vi "CC Quad Image Viewer.vi"(11 "Files":path[](array[path])) -> ()   [LabVIEW 2024]
uses:
  <vilib>/Utility/miscctls.llb/LVCursorListTypeDef.ctl
panel:
  in  "Transpose 1":bool
  out "Detector 1":sgl[][](graph)
  in  "Transpose 2":bool
  out "Detector 2":sgl[][](graph)
  in  "Transpose 3":bool
  out "Detector 3":sgl[][](graph)
  in  "Transpose 4":bool
  out "Detector 4":sgl[][](graph)
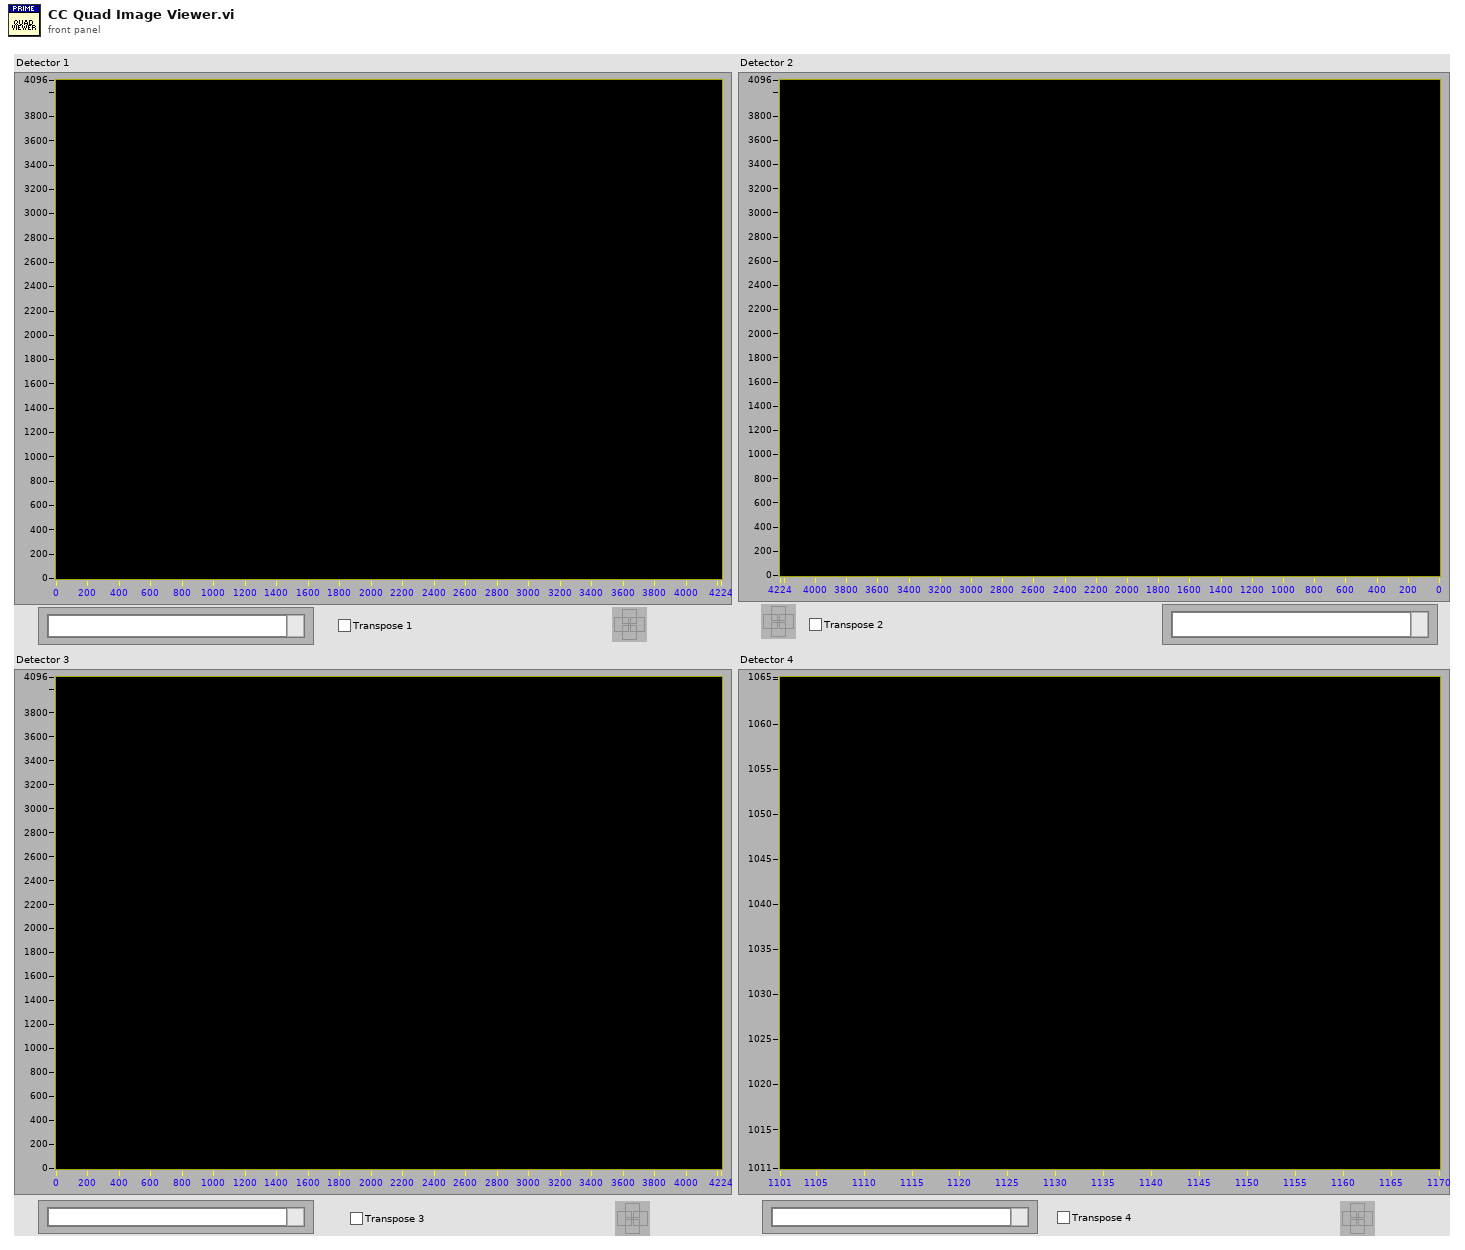
[diagram p1: front panel]
types:
  T1 = cluster{"state":refnum<user-event>, "plots":refnum<vi>[]}
  T2 = typedef "LVCursorListTypeDef.ctl" = cluster{"Name":string, "Color":u32, "Style":u8, "Point Style":u8, "Name Visible":bool, "Allow Drag":bool, "Cursor Mode":u32, "Plot":i32, "Index":i32, "Position":cluster{"X":dbl, "Y":dbl}, "X Scale":u32, "Y Scale":u32, "Watch Plots":i32[], "Watch All Plots":bool, "Plot Area":i32, "Label Offset":cluster{"X":dbl, "Y":dbl}}[]
  T3 = typedef "LVRectTypeDef.ctl" = cluster{"Left":i16, "Top":i16, "Right":i16, "Bottom":i16}
  T4 = typedef "CC cluster  Viewer Image Order.ctl" = cluster{"Top Left":i32, "Top Right":i32, "Bottom Left":i32, "Bottom Right":i32}
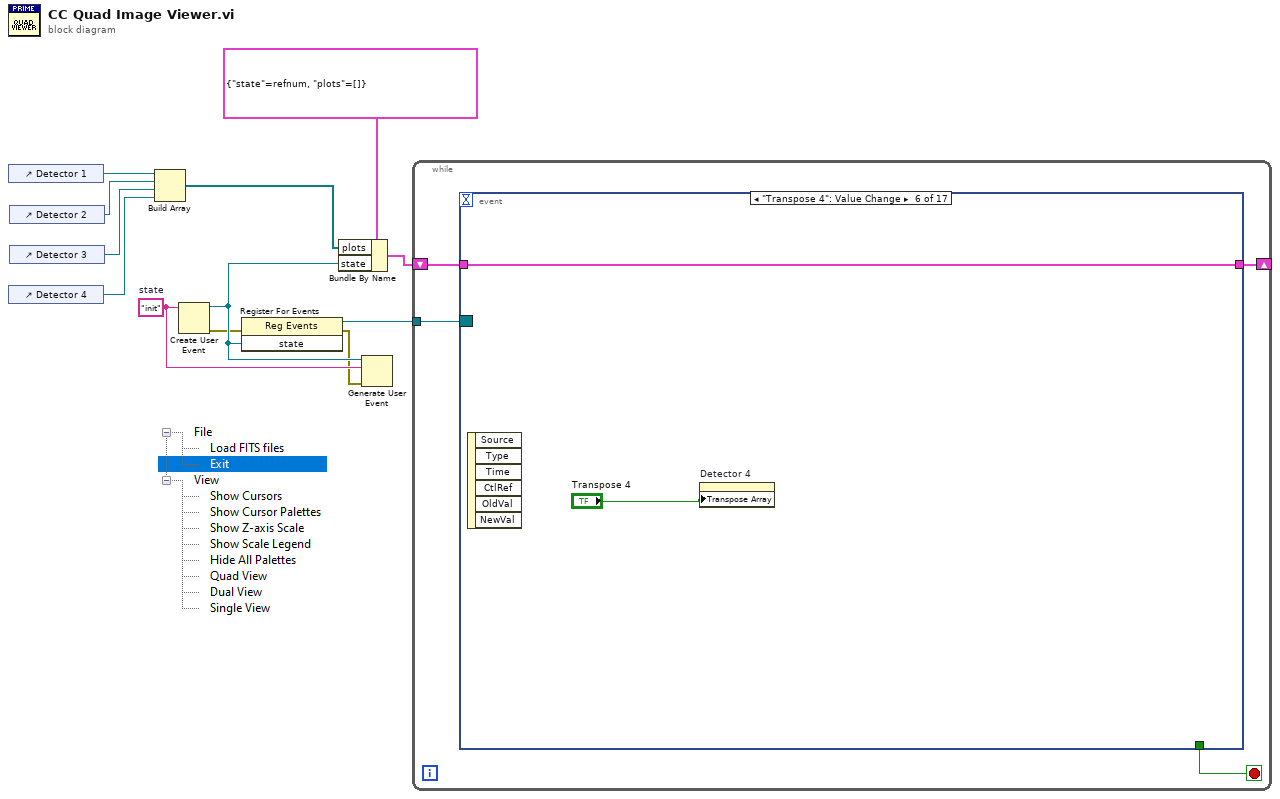
[diagram p0: block diagram]
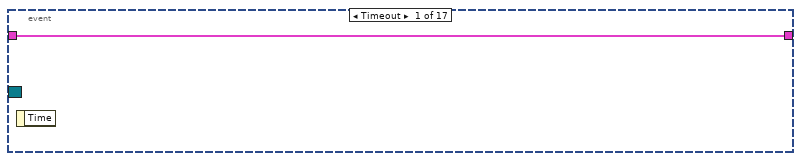
[diagram p2: hidden frame]
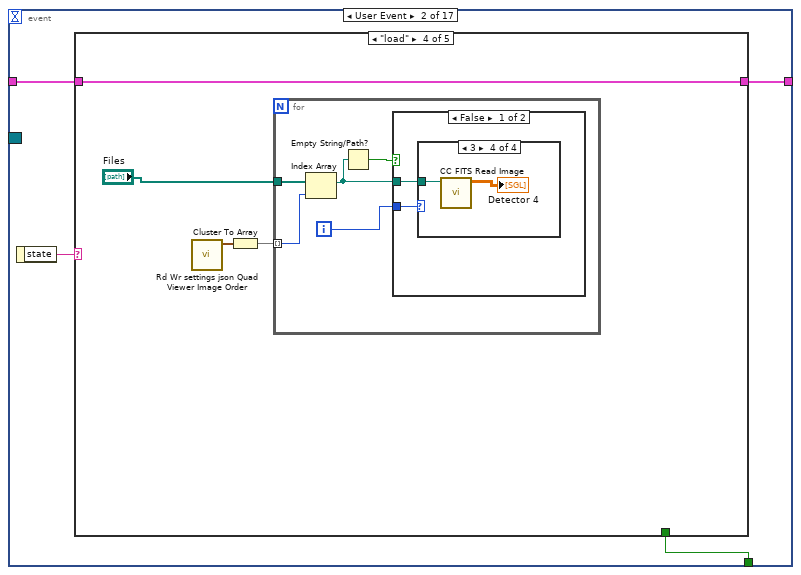
[diagram p3: hidden frame]
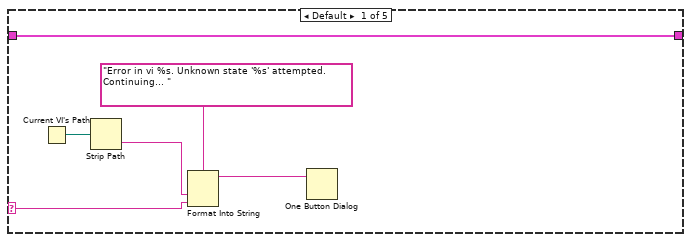
[diagram p4: hidden frame]
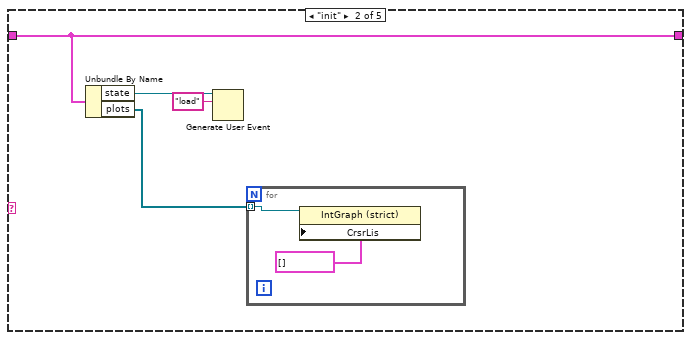
[diagram p5: hidden frame]
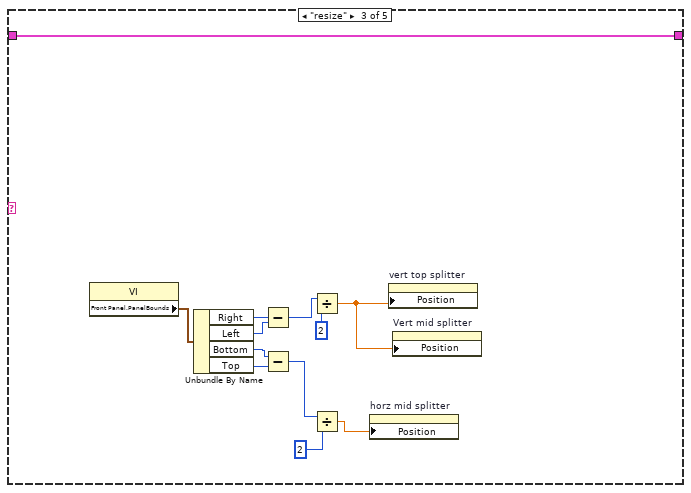
[diagram p6: hidden frame]
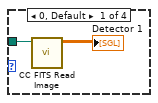
[diagram p7: hidden frame]
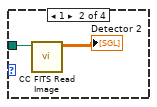
[diagram p8: hidden frame]
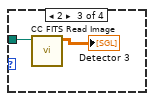
[diagram p9: hidden frame]
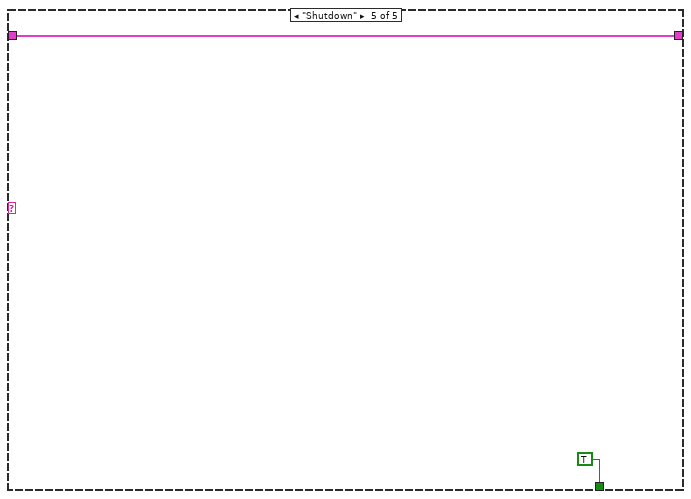
[diagram p11: hidden frame]
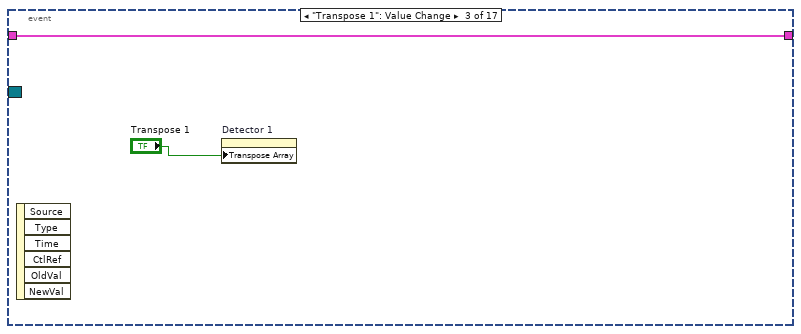
[diagram p12: hidden frame]
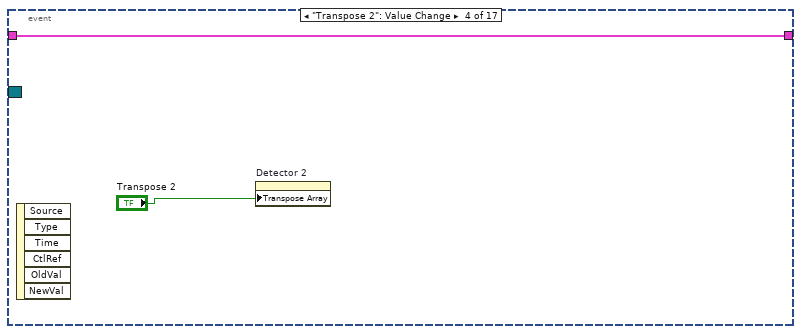
[diagram p13: hidden frame]
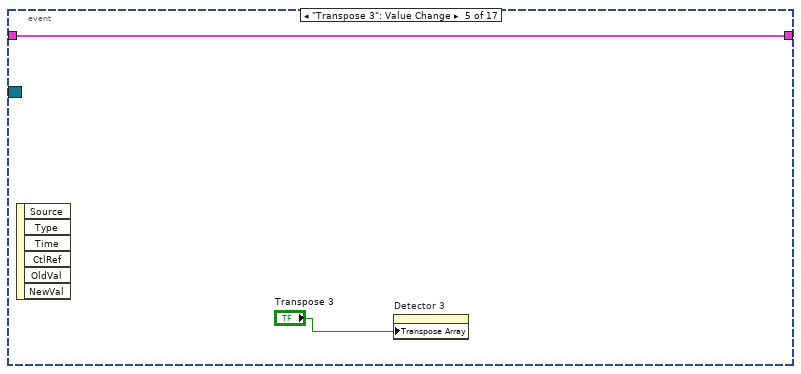
[diagram p14: hidden frame]
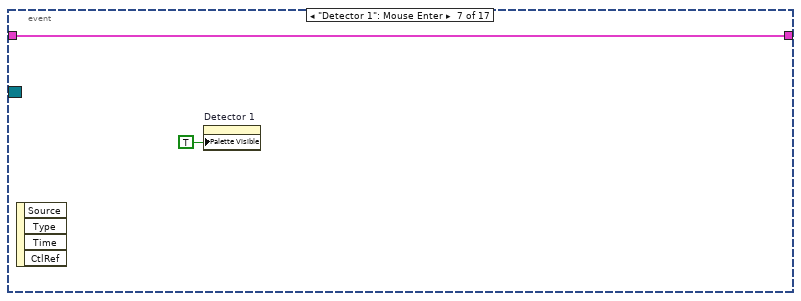
[diagram p15: hidden frame]
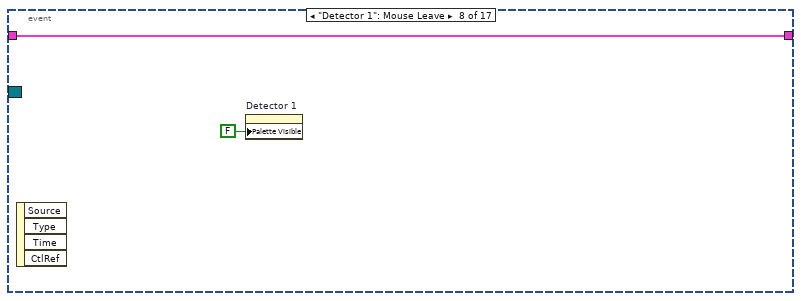
[diagram p16: hidden frame]
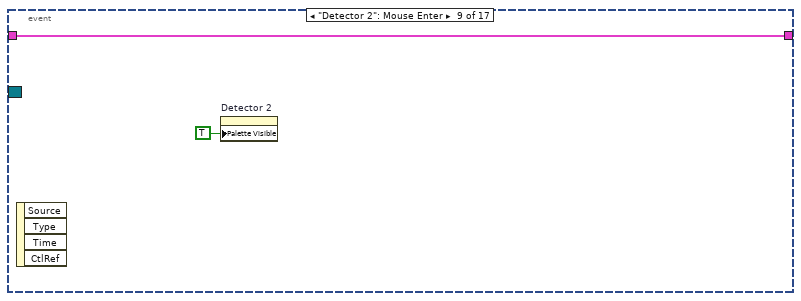
[diagram p17: hidden frame]
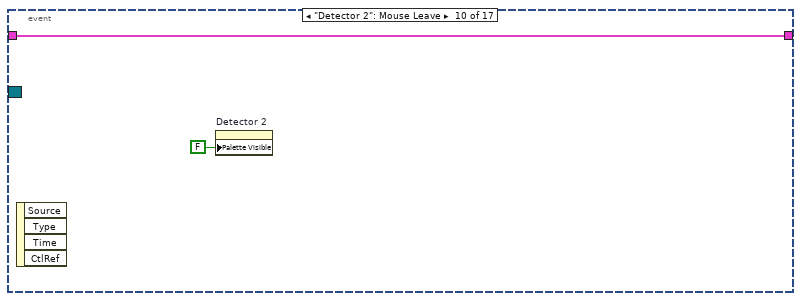
[diagram p18: hidden frame]
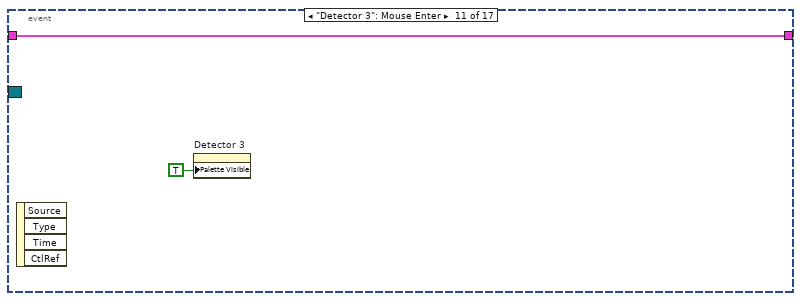
[diagram p19: hidden frame]
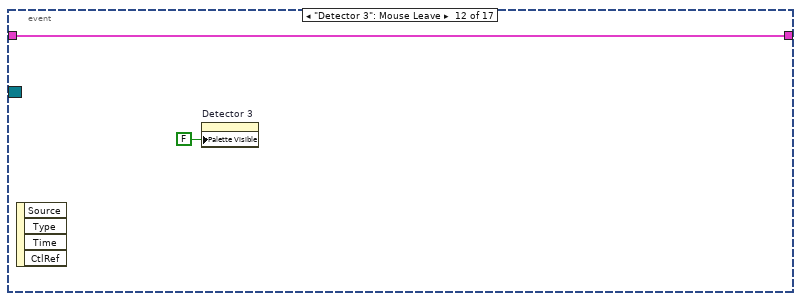
[diagram p20: hidden frame]
diagram:
  w8 = "init"  # state
  n1 = control-ref of="Detector 1"() -> (w5:refnum<vi>)
  n2 = control-ref of="Detector 4"() -> (w2:refnum<vi>)
  n3 = control-ref of="Detector 2"() -> (w4:refnum<vi>)
  n4 = control-ref of="Detector 3"() -> (w3:refnum<vi>)
  n5 = Build Array(w5, w4, w3, w2) -> (w1:refnum<vi>[])
  n6 = Create User Event(user event datatype=w8) -> (user event=w10:refnum<user-event>, error out=w6:errorcluster)  [unwired: 1 in]
  n7 = register-events(error in=w6, w10) -> (reference out=w9:refnum<event-registration>, error out=w7:errorcluster)  [unwired: 1 in]
  n8 = Bundle By Name(cluster=T1 {"state"=refnum, "plots"=[]}, "plots"=w1, "state"=w10) -> (w11:T1)
  n9 = Generate User Event(user event=w10, event data cluster=w8, error in=w7) -> ()  [unwired: 1 in, 2 out]
  n10 = while {
    tunnel: w9 -> [w16]
    shift-right: [w14] -> _
    shift-left: w11 -> [w15]
    stop <- w13 stop-if-true
    n11 = event shown="[5] \"Transpose 4\": Value Change" {
      selector: w16 -> [_ _ _ _ _ _ _ _ _ _ _ _ _ _ _ _ _]
      dyn-events: _ -> [_ _ _ _ _ _ _ _ _ _ _ _ _ _ _ _ _]
      timeout: _ -> [_ _ _ _ _ _ _ _ _ _ _ _ _ _ _ _ _]
      tunnel: w15 -> [w17 w20 w68 w70 w72 w74 w76 w78 w80 w82 w84 w86 w88 w90 w94 w151 w155]
      tunnel: [w17 w19 w68 w70 w72 w74 w76 w78 w80 w82 w84 w86 w88 w90 w94 w151 w155] -> w14
      tunnel: [_ w18 _ _ _ _ _ _ _ _ _ _ _ _ _ _ _] -> w13
      event Timeout {
        n12 = event-data() -> ()  [unwired: 1 in, 1 out]
      }
      event User Event {
        n13 = event-data() -> ("state"=w21:string)  [unwired: 1 in]
        n14 = case shown="\"load\"" w21 {
          selector: w21 -> [w26 _ _ _ _]
          tunnel: w20 -> [w22 w31 w45 w49 w66]
          tunnel: [w22 w31 w45 w49 w66] -> w19
          tunnel: [_ _ _ _ TRUE] -> w18
          frame Default {
            n15 = Current VI's Path() -> (path=w25:path)
            n16 = Strip Path(path=w25) -> (name=w24:string)  [unwired: 1 out]
            n17 = Format Into String(format string="Error in vi %s. Unknown state '%s' attempted. Continuing... ", w24, w26) -> (resulting string=w23:string)  [unwired: 2 in, 1 out]
            n18 = One Button Dialog(message=w23) -> ()  [unwired: 1 in, 1 out]
          }
          frame "init" {
            n19 = Unbundle By Name(w31) -> ("state"=w30:refnum<user-event>, "plots"=w28:refnum<vi>[])
            n20 = Generate User Event(user event=w30, event data cluster="load" ("event data")) -> ()  [unwired: 2 in, 2 out]
            n21 = for {
              tunnel: w28 -> [w33] mode=indexing
              n22 = property class="IntGraph (strict)"(reference=w33, "CrsrLis"=T2 [] ("Cursor List")) -> ()  [unwired: 1 in, 2 out]
            }
          }
          frame "resize" {
            n23 = property class="VI"() -> ("Front Panel.PanelBounds"=w42:T3)  [unwired: 2 in, 2 out]
            n24 = Unbundle By Name(w42) -> ("Right"=w39:i16, "Left"=w38:i16, "Bottom"=w35:i16, "Top"=w36:i16)
            n25 = Subtract(x=w39, y=w38) -> (x-y=w37:i16)
            n26 = Subtract(x=w35, y=w36) -> (x-y=w34:i16)
            n27 = Divide(x=w37, y=2) -> (x/y=w41:dbl)
            n28 = Divide(x=w34, y=2) -> (x/y=w40:dbl)
            n29 = property on="horz mid splitter" class="Splitter"("Position"=w40) -> ()  [unwired: 2 in, 2 out]
            n30 = property on="vert top splitter" class="Splitter"("Position"=w41) -> ()  [unwired: 2 in, 2 out]
            n31 = property on="Vert mid splitter" class="Splitter"("Position"=w41) -> ()  [unwired: 2 in, 2 out]
          }
          frame "load" {
            n32 = call "Rd Wr settings json Quad Viewer Image Order.vi"() -> ("Image Order"=w47:T4)  [unwired: 10 in, 1 out]
            n33 = Cluster To Array(cluster=w47) -> (array=w46:i32[])
            n34 = for {
              tunnel: "Files" -> [w53]
              tunnel: w46 -> [w52] mode=indexing
              i -> [w54]
              n35 = Index Array(array=w53, index=w52) -> (element=w51:path)
              n36 = Empty String/Path?(string/path=w51) -> (empty?=w50:bool)
              n37 = case shown="False" w50 {
                tunnel: w54 -> [w56 _]
                tunnel: w51 -> [w55 _]
                frame False {
                  n38 = case shown="3" w56 {
                    tunnel: w55 -> [w58 w60 w62 w64]
                    frame 0, Default {
                      n39 = call "CC FITS Read Image.vi"("FITS File Path"=w58) -> ("Image"=→"Detector 1":sgl[][])  [unwired: 9 in, 1 out]
                    }
                    frame 1 {
                      n40 = call "CC FITS Read Image.vi"("FITS File Path"=w60) -> ("Image"=→"Detector 2":sgl[][])  [unwired: 9 in, 1 out]
                    }
                    frame 2 {
                      n41 = call "CC FITS Read Image.vi"("FITS File Path"=w62) -> ("Image"=→"Detector 3":sgl[][])  [unwired: 9 in, 1 out]
                    }
                    frame 3 {
                      n42 = call "CC FITS Read Image.vi"("FITS File Path"=w64) -> ("Image"=→"Detector 4":sgl[][])  [unwired: 9 in, 1 out]
                    }
                  }
                }
                frame True {
                }
              }
            }
          }
          frame "Shutdown" {
          }
        }
      }
      event "Transpose 1": Value Change {
        n43 = event-data() -> ()  [unwired: 1 in, 6 out]
        n44 = property on="Detector 1" class="IntGraph (strict)"("Transpose Array"="Transpose 1") -> ()  [unwired: 2 in, 2 out]
      }
      event "Transpose 2": Value Change {
        n45 = event-data() -> ()  [unwired: 1 in, 6 out]
        n46 = property on="Detector 2" class="IntGraph (strict)"("Transpose Array"="Transpose 2") -> ()  [unwired: 2 in, 2 out]
      }
      event "Transpose 3": Value Change {
        n47 = event-data() -> ()  [unwired: 1 in, 6 out]
        n48 = property on="Detector 3" class="IntGraph (strict)"("Transpose Array"="Transpose 3") -> ()  [unwired: 2 in, 2 out]
      }
      event "Transpose 4": Value Change {
        n49 = event-data() -> ()  [unwired: 1 in, 6 out]
        n50 = property on="Detector 4" class="IntGraph (strict)"("Transpose Array"="Transpose 4") -> ()  [unwired: 2 in, 2 out]
      }
      event "Detector 1": Mouse Enter {
        n51 = event-data() -> ()  [unwired: 1 in, 4 out]
        n52 = property on="Detector 1" class="IntGraph (strict)"("Palette Visible"=TRUE ("Palette:Visible")) -> ()  [unwired: 2 in, 2 out]
      }
      event "Detector 1": Mouse Leave {
        n53 = event-data() -> ()  [unwired: 1 in, 4 out]
        n54 = property on="Detector 1" class="IntGraph (strict)"("Palette Visible"=FALSE ("Palette:Visible")) -> ()  [unwired: 2 in, 2 out]
      }
      event "Detector 2": Mouse Enter {
        n55 = event-data() -> ()  [unwired: 1 in, 4 out]
        n56 = property on="Detector 2" class="IntGraph (strict)"("Palette Visible"=TRUE ("Palette:Visible")) -> ()  [unwired: 2 in, 2 out]
      }
      event "Detector 2": Mouse Leave {
        n57 = event-data() -> ()  [unwired: 1 in, 4 out]
        n58 = property on="Detector 2" class="IntGraph (strict)"("Palette Visible"=FALSE ("Palette:Visible")) -> ()  [unwired: 2 in, 2 out]
      }
      event "Detector 3": Mouse Enter {
        n59 = event-data() -> ()  [unwired: 1 in, 4 out]
        n60 = property on="Detector 3" class="IntGraph (strict)"("Palette Visible"=TRUE ("Palette:Visible")) -> ()  [unwired: 2 in, 2 out]
      }
      event "Detector 3": Mouse Leave {
        n61 = event-data() -> ()  [unwired: 1 in, 4 out]
        n62 = property on="Detector 3" class="IntGraph (strict)"("Palette Visible"=FALSE ("Palette:Visible")) -> ()  [unwired: 2 in, 2 out]
      }
      event "Detector 4": Mouse Enter {
        n63 = event-data() -> ()  [unwired: 1 in, 4 out]
        n64 = property on="Detector 4" class="IntGraph (strict)"("Palette Visible"=TRUE ("Palette:Visible")) -> ()  [unwired: 2 in, 2 out]
      }
      event "Detector 4": Mouse Leave {
        n65 = event-data() -> ()  [unwired: 1 in, 4 out]
        n66 = property on="Detector 4" class="IntGraph (strict)"("Palette Visible"=FALSE ("Palette:Visible")) -> ()  [unwired: 2 in, 2 out]
      }
      event Menu Selection (User) {
        n67 = event-data() -> ("MenuRef"=w92:refnum<k9>, "ItemTag"=w95:string)  [unwired: 1 in, 5 out]
        n68 = Unbundle By Name(w94) -> ("state"=w91:refnum<user-event>, "plots"=w93:refnum<vi>[])
        n69 = case shown="\"Show Cursor Palettes\"" w95 {
          selector: w95 -> [_ w98 w114 w123 w132 w141 _]
          tunnel: w93 -> [_ w101 w111 w120 w129 w138 _]
          tunnel: w92 -> [_ w97 w115 w124 w133 w144 _]
          tunnel: w91 -> [_ _ _ _ _ _ w149]
          frame "False", Default {
          }
          frame "Show Cursors" {
            n70 = Get Menu Item Info(7:w98, 11:w97) -> (3:w100:refnum<k9>, 4:w99:bool)  [unwired: 1 in, 5 out]
            n71 = Not(x=w99) -> (.not. x?=w96:bool)
            n72 = for {
              tunnel: w101 -> [w106] mode=indexing
              tunnel: w96 -> [w102]
              n73 = property class="IntGraph (strict)"(reference=w106) -> (reference out=w103:refnum<vi>, "CrsrLis"=w105:T2)  [unwired: 1 in, 1 out]
              n74 = Array Size(array=w105) -> (size(s)=w104:i32)
              n75 = for {
                N: w104 -> [_]
                tunnel: w103 -> [w109]
                tunnel: w102 -> [w107]
                i -> [w108]
                n76 = property class="IntGraph (strict)"(reference=w109, "Active Cursor"=w108, "Cursor.Visible"=w107) -> ()  [unwired: 1 in, 2 out]
              }
            }
            n77 = Set Menu Item Info(6:w96, 7:w98, 11:w100) -> ()  [unwired: 4 in, 2 out]
          }
          frame "Show Cursor Palettes" {
            n78 = Get Menu Item Info(7:w114, 11:w115) -> (3:w113:refnum<k9>, 4:w112:bool)  [unwired: 1 in, 5 out]
            n79 = Not(x=w112) -> (.not. x?=w110:bool)
            n80 = for {
              tunnel: w111 -> [w118] mode=indexing
              tunnel: w110 -> [w117]
              n81 = property class="IntGraph (strict)"(reference=w118, "Cursor Palette Vis"=w117) -> (reference out=w116:refnum<vi>)  [unwired: 1 in, 1 out]
              n82 = invoke class="IntGraph (strict)" method="FitControlToPane"(reference=w116) -> ()  [unwired: 2 in, 3 out]
            }
            n83 = Set Menu Item Info(6:w110, 7:w114, 11:w113) -> ()  [unwired: 4 in, 2 out]
          }
          frame "Show Z-axis Scale" {
            n84 = Get Menu Item Info(7:w123, 11:w124) -> (3:w122:refnum<k9>, 4:w121:bool)  [unwired: 1 in, 5 out]
            n85 = Not(x=w121) -> (.not. x?=w119:bool)
            n86 = for {
              tunnel: w120 -> [w127] mode=indexing
              tunnel: w119 -> [w126]
              n87 = property class="IntGraph (strict)"(reference=w127, "ZScale.Visible"=w126, "ZScale.RampVis"=w126) -> (reference out=w125:refnum<vi>)  [unwired: 1 in, 1 out]
              n88 = invoke class="IntGraph (strict)" method="FitControlToPane"(reference=w125) -> ()  [unwired: 2 in, 3 out]
            }
            n89 = Set Menu Item Info(6:w119, 7:w123, 11:w122) -> ()  [unwired: 4 in, 2 out]
          }
          frame "Show Scale Legend" {
            n90 = Get Menu Item Info(7:w132, 11:w133) -> (3:w131:refnum<k9>, 4:w130:bool)  [unwired: 1 in, 5 out]
            n91 = Not(x=w130) -> (.not. x?=w128:bool)
            n92 = for {
              tunnel: w129 -> [w136] mode=indexing
              tunnel: w128 -> [w135]
              n93 = property class="IntGraph (strict)"(reference=w136, "ScaleLegendVis"=w135) -> (reference out=w134:refnum<vi>)  [unwired: 1 in, 1 out]
              n94 = invoke class="IntGraph (strict)" method="FitControlToPane"(reference=w134) -> ()  [unwired: 2 in, 3 out]
            }
            n95 = Set Menu Item Info(6:w128, 7:w132, 11:w131) -> ()  [unwired: 4 in, 2 out]
          }
          frame "Hide All Palettes" {
            n96 = Get Menu Item Info(7:w141, 11:w144) -> (2:w142:string, 3:w143:refnum<k9>)  [unwired: 1 in, 5 out]
            n97 = Not Equal?(x=w141, y=w142) -> (x != y?=w137:bool)
            n98 = for {
              tunnel: w138 -> [w147] mode=indexing
              tunnel: w137 -> [w145]
              n99 = property class="IntGraph (strict)"(reference=w147, "ScaleLegendVis"=w145, "ZScale.Visible"=w145, "ZScale.RampVis"=w145, "ScaleLegendVis"=w145, "Cursor Palette Vis"=w145, "Palette Visible"=w145) -> (reference out=w146:refnum<vi>)  [unwired: 1 in, 1 out]
              n100 = invoke class="IntGraph (strict)" method="FitControlToPane"(reference=w146) -> ()  [unwired: 2 in, 3 out]
            }
            n101 = Select(t=w141, s=w137, f="Show Palettes") -> (s? t:f=w140:string)
            n102 = Set Menu Item Info(7:w141, 10:w140, 11:w143) -> ()  [unwired: 4 in, 2 out]
          }
          frame "Exit" {
            n103 = Generate User Event(user event=w149, event data cluster="Shutdown" ("event data")) -> ()  [unwired: 2 in, 2 out]
          }
        }
      }
      event Panel Close {
        n104 = event-data() -> ()  [unwired: 1 in, 4 out]
        n105 = Unbundle By Name(w151) -> ("state"=w150:refnum<user-event>)
        n106 = Generate User Event(user event=w150, event data cluster="Shutdown" ("event data")) -> ()  [unwired: 2 in, 2 out]
      }
      event Panel Resize {
        n107 = event-data() -> ()  [unwired: 1 in, 8 out]
        n108 = Unbundle By Name(w155) -> ("state"=w154:refnum<user-event>)
        n109 = Generate User Event(user event=w154, event data cluster="resize" ("event data")) -> ()  [unwired: 2 in, 2 out]
      }
    }
  }
